vi "CleanUpData.vi"(0 "VIA CFG Data":T1 {"Test Configuration"."Test Ranking" items=["Low", "Normal", "High"]}, 11 "Error In":errorcluster) -> (4 "VIA CFG Data":T1 {"Test Configuration"."Test Ranking" items=["Low", "Normal", "High"]}, 15 "Error Out":errorcluster)   [LabVIEW 2020]
uses:
  <vilib>/addons/analyzer/Typedefs/VIACFGExport.ctl
  <vilib>/addons/analyzer/_analyzerctrls.llb/VIAnCtl TestRanking.ctl
  <vilib>/addons/analyzer/_analyzerctrls.llb/VIAnCtl Config Control Value.ctl
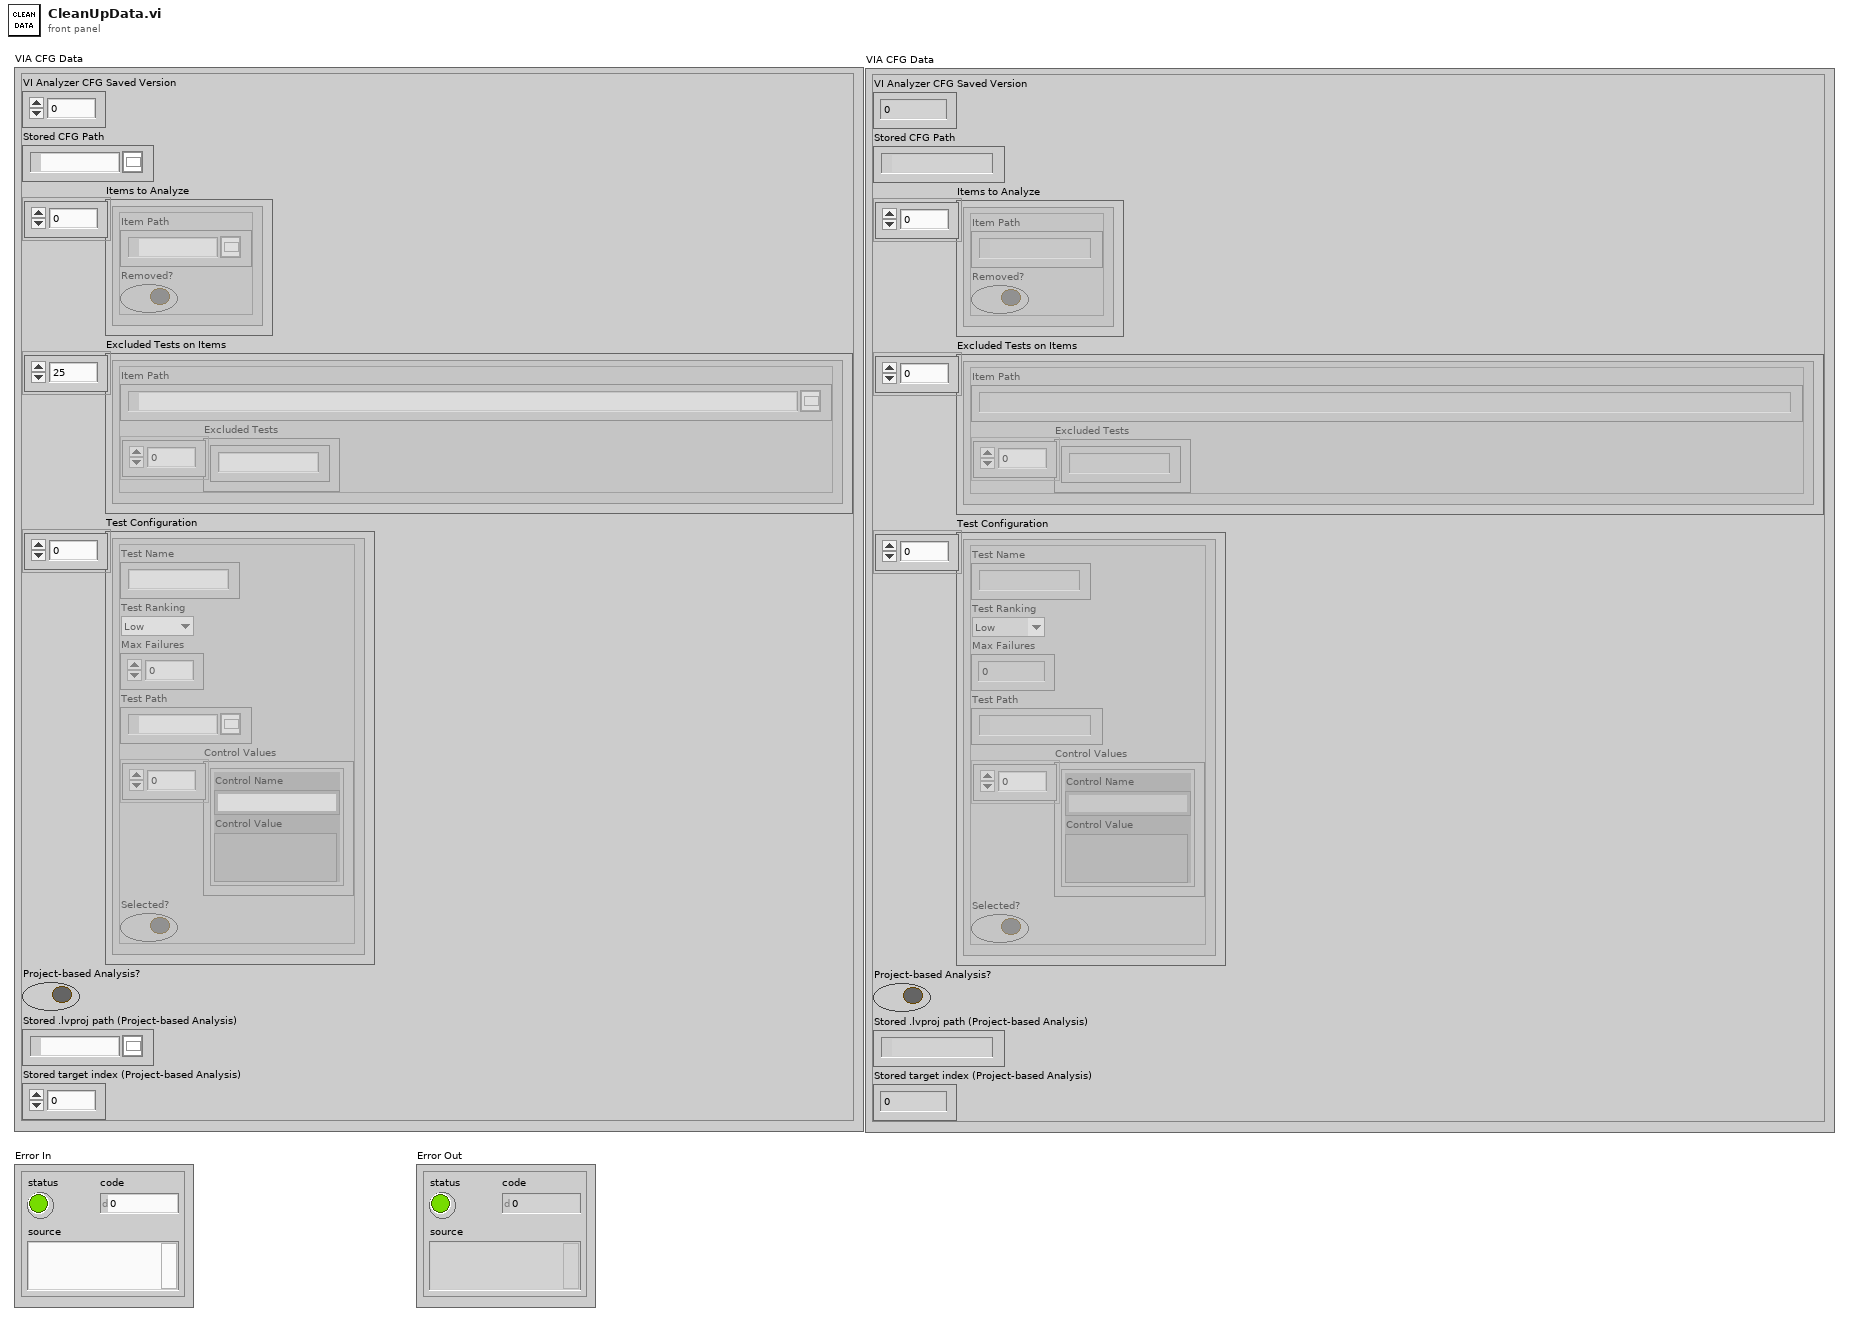
[diagram p1: front panel]
types:
  T1 = typedef "VIACFGExport.ctl" = cluster{"VI Analyzer CFG Saved Version":u16, "Stored CFG Path":path, "Items to Analyze":cluster{"Item Path":path, "Removed?":bool}[], "Excluded Tests on Items":cluster{"Item Path":path, "Excluded Tests":string[]}[], "Test Configuration":cluster{"Test Name":string, "Test Ranking":T2, "Max Failures":u32, "Test Path":path, "Control Values":T3[], "Selected?":bool}[], "Project-based Analysis?":bool, "Stored .lvproj path (Project-based Analysis)":path, "Stored target index (Project-based Analysis)":u16}
  T2 = typedef "VIAnCtl TestRanking.ctl" = u16
  T3 = typedef "VIAnCtl Config Control Value.ctl" = cluster{"Control Name":string, "Control Value":variant}
  T4 = cluster{"Item Path":path, "Excluded Tests":string[]}[]
  T5 = cluster{"Item Path":path, "Excluded Tests":string[]}
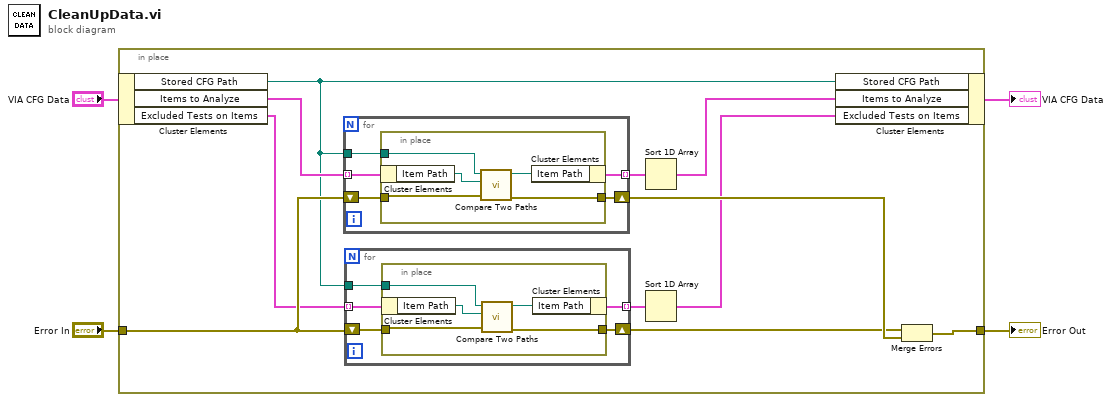
[diagram p0: block diagram]
diagram:
  n1 = in-place {
    in-place-border: "Error In" -> [w12]
    in-place-border: [w11] -> w3
    n2 = in-place-cluster #1("VIA CFG Data") -> ("Stored CFG Path"=w9:path, "Items to Analyze"=w14:cluster{"Item Path":path, "Removed?":bool}[], "Excluded Tests on Items"=w5:T4)
    n3 = for {
      tunnel: w14 -> [w27] mode=indexing
      tunnel: w9 -> [w30]
      shift-right: [w28] -> w15
      shift-left: w12 -> [w29]
      tunnel: [w26] -> w7 mode=indexing
      n4 = in-place {
        in-place-border: w30 -> [w35]
        in-place-border: w29 -> [w34]
        in-place-border: [w33] -> w28
        n5 = in-place-cluster #2(w27) -> ("Item Path"=w32:path)
        n6 = call <vilib>:"Compare Two Paths.vi"("error in (no error)"=w34, "Path 2"=w32, "Path 1"=w35) -> ("error out"=w33:errorcluster, "Relative Path from 1 to 2"=w31:path)  [unwired: 5 in, 2 out]
        n7 = in-place-cluster #2("Item Path"=w31) -> (w26:cluster{"Item Path":path, "Removed?":bool})
      }
    }
    n8 = for {
      tunnel: w5 -> [w17] mode=indexing
      tunnel: w9 -> [w20]
      shift-right: [w18] -> w10
      shift-left: w12 -> [w19]
      tunnel: [w16] -> w6 mode=indexing
      n9 = in-place {
        in-place-border: w20 -> [w25]
        in-place-border: w19 -> [w24]
        in-place-border: [w23] -> w18
        n10 = in-place-cluster #3(w17) -> ("Item Path"=w22:path)
        n11 = call <vilib>:"Compare Two Paths.vi"("error in (no error)"=w24, "Path 2"=w22, "Path 1"=w25) -> ("error out"=w23:errorcluster, "Relative Path from 1 to 2"=w21:path)  [unwired: 5 in, 2 out]
        n12 = in-place-cluster #3("Item Path"=w21) -> (w16:T5)
      }
    }
    n13 = Sort 1D Array(array=w7) -> (sorted array=w13:cluster{"Item Path":path, "Removed?":bool}[])
    n14 = Sort 1D Array(array=w6) -> (sorted array=w8:T4)
    n15 = in-place-cluster #1("Stored CFG Path"=w9, "Items to Analyze"=w13, "Excluded Tests on Items"=w8) -> (→"VIA CFG Data":T1)
    n16 = Merge Errors(w10, w15) -> (w11:errorcluster)
  }
  "Error Out" <- w3
